vi "read_attributes.vi"(8 "error in (no error)":errorcluster, 11 "SpectralEmbedding in":refnum<class "SpectralEmbedding.lvclass">) -> (0 "error out":errorcluster, 2 "attributes":T1, 3 "SpectralEmbedding out":refnum<class "SpectralEmbedding.lvclass">)   [LabVIEW 2020, in "SpectralEmbedding.lvclass"]
uses:
  SpectralEmbedding.lvclass
  Controls/spectral_embedding_attributes.ctl
  SpectralEmbedding.lvclass/SpectralEmbedding.ctl
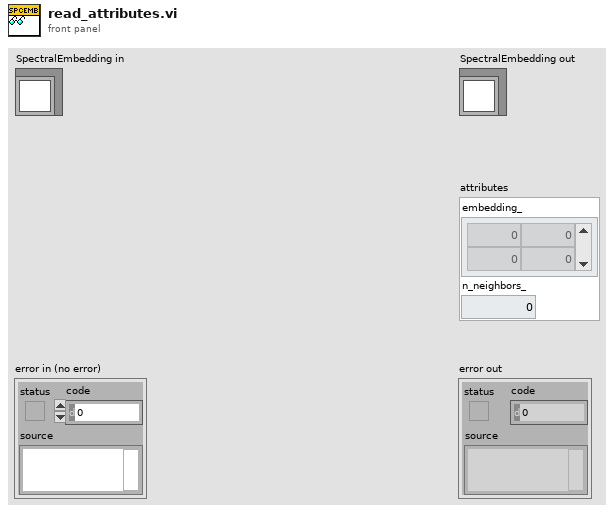
[diagram p1: front panel]
types:
  T1 = typedef "spectral_embedding_attributes.ctl" = cluster{"embedding_":dbl[][], "n_neighbors_":dbl}
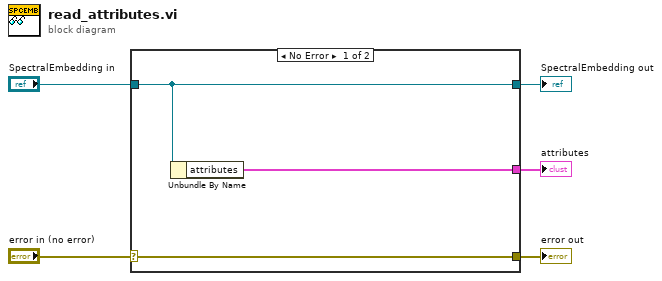
[diagram p0: block diagram]
diagram:
  n1 = case shown="No Error" "error in (no error)" {
    selector: "error in (no error)" -> [w8 w9]
    tunnel: [w8 w9] -> w4
    tunnel: [w7 w10] -> w2
    tunnel: "SpectralEmbedding in" -> [w7 w10]
    tunnel: [w6 _] -> w1
    frame No Error {
      n2 = Unbundle By Name(w7) -> ("attributes"=w6:T1)
    }
    frame Error {
    }
  }
  "error out" <- w4
  "SpectralEmbedding out" <- w2
  "attributes" <- w1
